vi "temp_function (SubVI).vi"(0 "Water state IN":i32, 2 "Temp IN":i32) -> (1 "Ready":bool=TRUE, 3 "Water state OUT":i32, 4 "Temp OUT":i32)   [LabVIEW 2018]
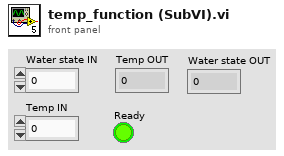
[diagram p1: front panel]
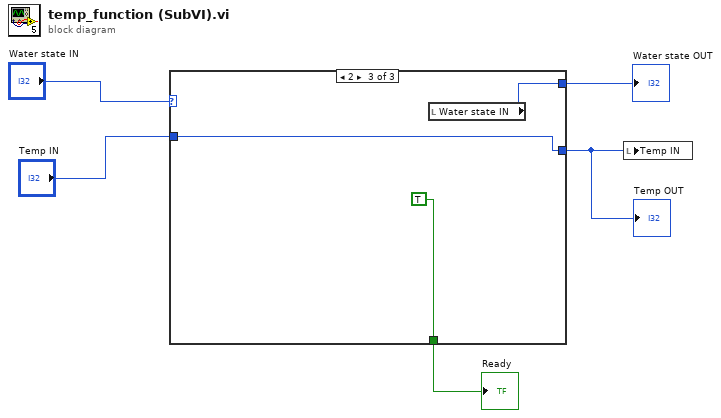
[diagram p0: block diagram]
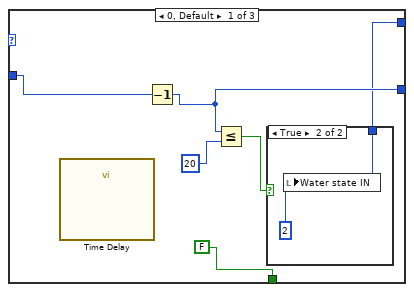
[diagram p2: hidden frame]
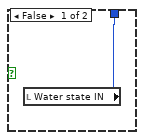
[diagram p3: hidden frame]
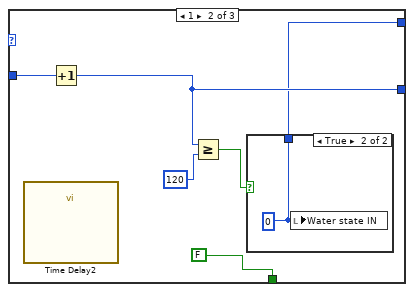
[diagram p4: hidden frame]
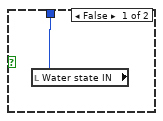
[diagram p5: hidden frame]
diagram:
  n1 = case shown="2" "Water state IN" {
    tunnel: "Temp IN" -> [w11 w19 w23]
    tunnel: [FALSE FALSE TRUE] -> w4
    tunnel: [w7 w15 w23] -> w2
    tunnel: [w6 w14 w22] -> w1
    frame 0, Default {
      n2 = call "Time Delay"() -> ()  [unwired: 11 in, 1 out]
      n3 = Decrement(x=w11) -> (x-1=w7:i32)
      n4 = Less Or Equal?(x=w7, y=20) -> (x <= y?=w9:bool)
      n5 = case shown="True" w9 {
        tunnel: [w12 w13] -> w6
        frame False {
          n6 = local read "Water state IN"() -> (w12:i32)
        }
        frame True {
          w13 = 2
          n7 = local write "Water state IN"(w13) -> ()
        }
      }
    }
    frame 1 {
      n8 = call "Time Delay2"() -> ()  [unwired: 11 in, 1 out]
      n9 = Increment(x=w19) -> (x+1=w15:i32)
      n10 = Greater Or Equal?(x=w15, y=120) -> (x >= y?=w18:bool)
      n11 = case shown="True" w18 {
        tunnel: [w20 w21] -> w14
        frame False {
          n12 = local read "Water state IN"() -> (w20:i32)
        }
        frame True {
          w21 = 0
          n13 = local write "Water state IN"(w21) -> ()
        }
      }
    }
    frame 2 {
      n14 = local read "Water state IN"() -> (w22:i32)
    }
  }
  "Ready" <- w4
  "Temp OUT" <- w2
  "Water state OUT" <- w1
  n15 = local write "Temp IN"(w2) -> ()
